vi "CS_cRIO-PB_DP-Slave_ReadWrite.vi"(0 "FPGA VI Reference":T2, 2 "Mode":T1(ring), 7 "Data":u8[](array[numeric]) format="%.0x", 11 "Error":errorcluster) -> (4 "FPGA VI Reference out":T2, 8 "Data out":u8[](array[numeric]) format="%.0x", 10 "Status":u8 format="%.0x", 15 "Error out":errorcluster)   [LabVIEW 2013, in "dynamic profibus.lvlib"]
uses:
  dynamic profibus.lvlib
  CS_cRIO-PB_DP-Slave_FPGA-Reference.ctl
  <vilib>/rvi/interface/common/niFpgaWaitOnOcc.vi
  <vilib>/Utility/error.llb/Error Cluster From Error Code.vi
  <vilib>/rvi/errors/niLvFpgaAdjustHostInterfaceError.vi
  <vilib>/rvi/interface/nirviReadWriteControl/nirviReadWriteControl.xnode
  NiFpgaLv.dll
  <vilib>/rvi/interface/Simulation/niFpgaSimulationCallBeginRW.vi
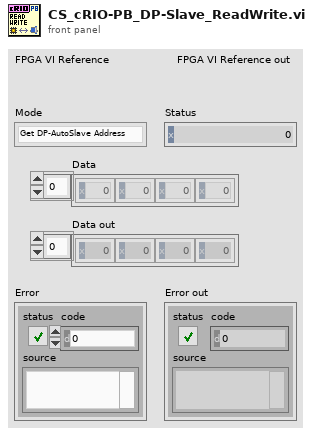
[diagram p1: front panel]
types:
  T1 = enum16{"Get DP-AutoSlave Address", "Set DP-AutoSlave Address", "Get Slave Output Data", "Set Slave Input Data", "Read/Write Slave Data"}
  T2 = typedef "dynamic profibus.lvlib/CS_cRIO-PB_DP-Slave_FPGA-Reference.ctl" = refnum<k20>
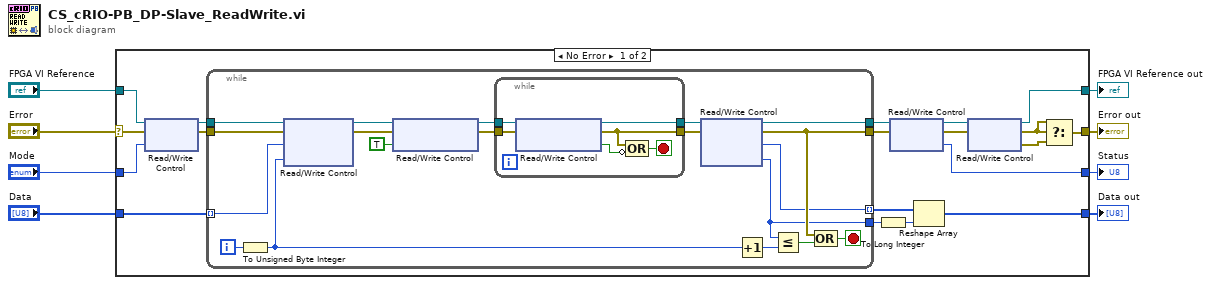
[diagram p0: block diagram]
diagram:
  n1 = case shown="No Error" "Error" {
    selector: "Error" -> [w27 w55]
    tunnel: "FPGA VI Reference" -> [w26 w54]
    tunnel: [w19 w55] -> w6
    tunnel: [w20 w54] -> w5
    tunnel: [w25 _] -> w4
    tunnel: "Mode" -> [w9 _]
    tunnel: "Data" -> [w14 w53]
    tunnel: [w11 w53] -> w2
    frame No Error {
      n2 = xnode "Read/Write Control"("FPGA VI Reference In"=w26, "error in"=w27, "Mode"=w9) -> ("FPGA VI Reference Out"=w15:T2, "error out"=w16:errorcluster)
      n3 = while {
        tunnel: w15 -> [w46]
        tunnel: [w38] -> w17
        tunnel: w16 -> [w37]
        tunnel: w14 -> [w35] mode=indexing
        tunnel: [w34] -> w18
        tunnel: [w29] -> w12
        tunnel: [w28] -> w10 mode=indexing
        i -> [w33]
        stop <- w39 stop-if-true
        n4 = To Unsigned Byte Integer(number=w33) -> (unsigned 8bit integer=w30:u8)
        n5 = xnode "Read/Write Control"("FPGA VI Reference In"=w46, "error in"=w37, "SetData"=w35, "ByteIndex"=w30) -> ("FPGA VI Reference Out"=w45:T2, "error out"=w44:errorcluster)
        n6 = xnode "Read/Write Control"("FPGA VI Reference In"=w45, "error in"=w44, "HostRequest"=TRUE ("GetData")) -> ("FPGA VI Reference Out"=w42:T2, "error out"=w43:errorcluster)
        n7 = while {
          tunnel: w43 -> [w52]
          tunnel: w42 -> [w48]
          tunnel: [w49] -> w41
          tunnel: [w47] -> w40
          stop <- w50 stop-if-true
          n8 = xnode "Read/Write Control"("FPGA VI Reference In"=w48, "error in"=w52) -> ("FPGA VI Reference Out"=w47:T2, "error out"=w49:errorcluster, "HostRequest"=w51:bool)
          n9 = Compound Arithmetic op=OR(w49, invert w51) -> (w50:bool)
        }
        n10 = xnode "Read/Write Control"("FPGA VI Reference In"=w40, "error in"=w41) -> ("FPGA VI Reference Out"=w34:T2, "error out"=w38:errorcluster, "GetData"=w28:u8, "DataLen"=w29:u8)
        n11 = Increment(x=w30) -> (x+1=w32:u8)
        n12 = Less Or Equal?(x=w29, y=w32) -> (x <= y?=w31:bool)
        n13 = Compound Arithmetic op=OR(w38, w31) -> (w39:bool)
      }
      n14 = To Long Integer(number=w12) -> (32bit integer=w13:i32)
      n15 = xnode "Read/Write Control"("FPGA VI Reference In"=w18, "error in"=w17) -> ("FPGA VI Reference Out"=w21:T2, "error out"=w22:errorcluster, "Status"=w25:u8)
      n16 = Reshape Array(w10, w13) -> (w11:u8[])
      n17 = xnode "Read/Write Control"("FPGA VI Reference In"=w21, "error in"=w22) -> ("FPGA VI Reference Out"=w20:T2, "error out"=w24:errorcluster, "Error"=w23:errorcluster)
      n18 = Select(t=w24, s=w24, f=w23) -> (s? t:f=w19:errorcluster)
    }
    frame Error {
    }
  }
  "Error out" <- w6
  "FPGA VI Reference out" <- w5
  "Status" <- w4
  "Data out" <- w2
